vi "goToVf.vi"(9 "RobotModelAllInformation in":T1, 10 "firstCall?":bool, 11 "Robot in":refnum<class "Robot.lvclass">) -> (2 "RobotModelAllInformation out":T1, 3 "Robot out":refnum<class "Robot.lvclass">)   [LabVIEW 2020, in "Game.lvclass"]
uses:
  Game.lvclass
  Controls/RobotModel.ctl
  Controls/RobotModelAllInformation.ctl
  Controls/RobotModelTestCrashCase.ctl
  Robot_class/Robot.lvclass
  C:/RoboIME/SSL_AI/Object_class/Object.lvclass
  Robot_class/Robot.lvclass/Robot.ctl
  Object_class/Object.lvclass/Object.ctl
  <vilib>/Analysis/_algsub.llb/Real Vector Norm.vi
  Object_class/Read x.vi
  Object_class/Read y.vi
  Robot_class/Read est_v_tang.vi
  Robot_class/Write v_tang.vi
  Robot_class/Write v_norm.vi
  Robot_class/Write v_ang.vi
  <vilib>/Analysis/NI_AALPro.lvlib
panel:
  in  "RobotModel":T2
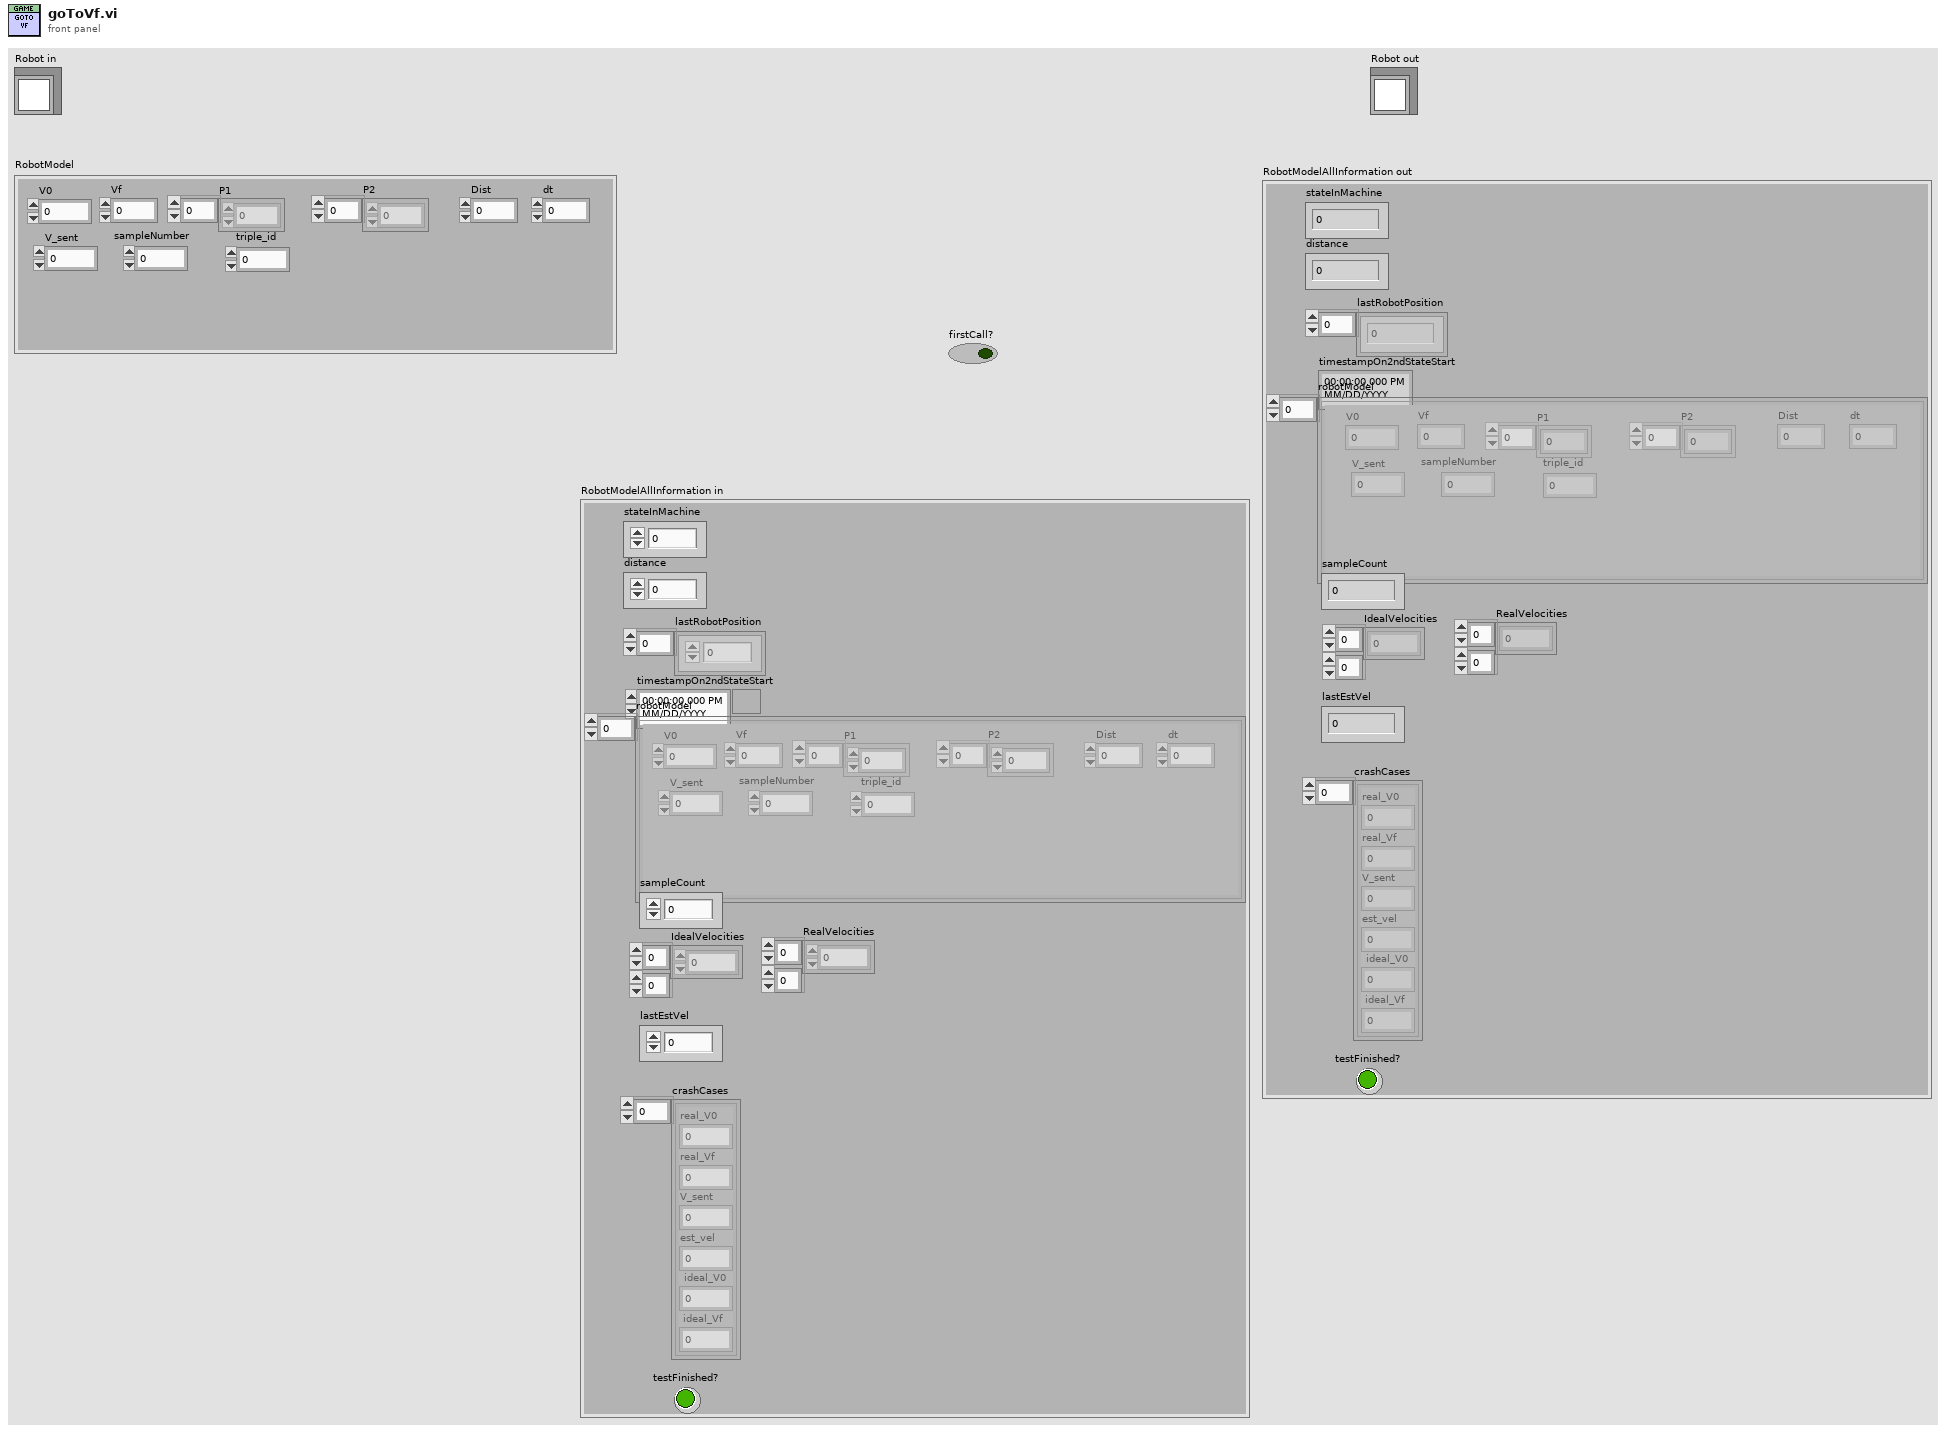
[diagram p1: front panel]
types:
  T1 = typedef "RobotModelAllInformation.ctl" = cluster{"distance":dbl, "lastRobotPosition":dbl[], "timestampOn2ndStateStart":timestamp, "robotModel":T2[], "sampleCount":i32, "stateInMachine":i32, "crashCases":T3[], "lastEstVel":dbl, "IdealVelocities":dbl[][], "RealVelocities":dbl[][], "testFinished?":bool}
  T2 = typedef "RobotModel.ctl" = cluster{"V0":dbl, "Vf":dbl, "Dist":dbl, "dt":dbl, "P1":dbl[], "P2":dbl[], "V_sent":dbl, "sampleNumber":i32, "triple_id":i32}
  T3 = typedef "RobotModelTestCrashCase.ctl" = cluster{"real_V0":dbl, "real_Vf":dbl, "V_sent":dbl, "est_vel":dbl, "ideal_V0":dbl, "ideal_Vf":dbl}
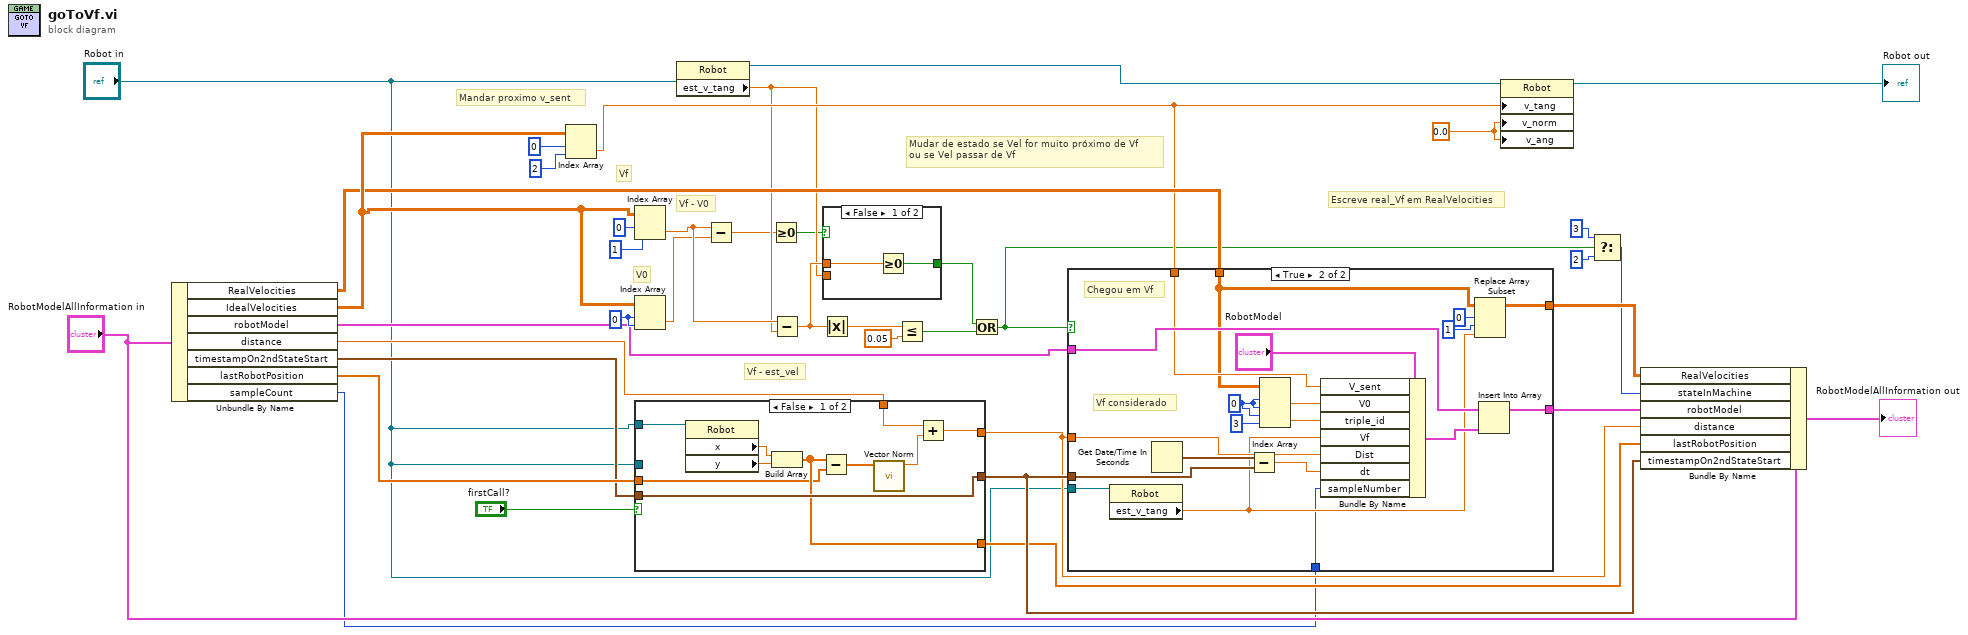
[diagram p0: block diagram]
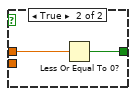
[diagram p2: hidden frame]
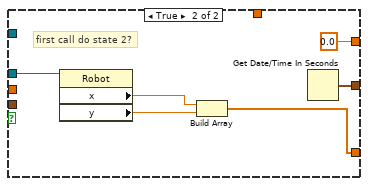
[diagram p4: hidden frame]
diagram:
  w38 = 0 ("index (row)")
  w3 = 0.0 ("v_norm")
  # "Escreve real_Vf em RealVelocities"
  # "Vf - est_vel"
  # "V0"
  # "Vf"
  # "Vf - V0"
  # "Mandar proximo v_sent"
  # "Mudar de estado se Vel for muito próximo de Vf\nou se Vel passar de Vf"
  n1 = Unbundle By Name("RobotModelAllInformation in") -> ("RealVelocities"=w29:dbl[][], "IdealVelocities"=w37:dbl[][], "robotModel"=w21:T2[], "distance"=w32:dbl, "timestampOn2ndStateStart"=w24:timestamp, "lastRobotPosition"=w30:dbl[], "sampleCount"=w1:i32)
  n2 = Index Array(array=w37, index (row)=0, index (col)=2 ("disabled index (col)")) -> (element=w28:dbl)
  n3 = Index Array(array=w37, index (row)=0, index (col)=1 ("disabled index (col)")) -> (element=w36:dbl)
  n4 = Index Array(array=w37, index (row)=w38, index (col)=w38) -> (element=w10:dbl)
  n5 = case shown="False" "firstCall?" {
    tunnel: [w49 w55] -> w33
    tunnel: w24 -> [w49 _]
    tunnel: "Robot in" -> [_ w54]
    tunnel: "Robot in" -> [w46 _]
    tunnel: [w40 0.0] -> w31
    tunnel: [w45 w51] -> w23
    tunnel: w30 -> [w43 _]
    tunnel: w32 -> [w42 _]
    frame False {
      n6 = property class="Robot"(reference=w46) -> ("x"=w47:dbl, "y"=w48:dbl)  [unwired: 1 in, 2 out]
      n7 = Build Array(w47, w48) -> (w45:dbl[])
      n8 = Subtract(x=w45, y=w43) -> (x-y=w44:dbl[])
      n9 = call-poly <vilib>:"Vector Norm.vi"("Input Vector"=w44) -> ("norm"=w41:dbl)  [unwired: 9 in, 1 out]
      n10 = Add(x=w42, y=w41) -> (x+y=w40:dbl)
    }
    frame True {
      # "first call do state 2?"
      n11 = property class="Robot"(reference=w54) -> ("x"=w53:dbl, "y"=w52:dbl)  [unwired: 1 in, 2 out]
      n12 = Build Array(w53, w52) -> (w51:dbl[])
      n13 = Get Date/Time In Seconds() -> (seconds since 1Jan1904=w55:timestamp)
    }
  }
  n14 = property class="Robot"(reference="Robot in") -> (reference out=w4:refnum<class "Robot.lvclass">, "est_v_tang"=w12:dbl)  [unwired: 1 in, 1 out]
  n15 = Subtract(x=w36, y=w10) -> (x-y=w7:dbl)
  n16 = Greater Or Equal To 0?(x=w7) -> (x >= 0?=w9:bool)
  n17 = Subtract(x=w36, y=w12) -> (x-y=w13:dbl)
  n18 = Absolute Value(x=w13) -> (abs(x)=w14:dbl)
  n19 = case shown="False" w9 {
    tunnel: [w57 w59] -> w16
    tunnel: w12 -> [_ _]
    tunnel: w13 -> [w56 w58]
    frame False {
      n20 = Greater Or Equal To 0?(x=w56) -> (x >= 0?=w57:bool)
    }
    frame True {
      n21 = Less Or Equal To 0?(x=w58) -> (x <= 0?=w59:bool)
    }
  }
  n22 = Less Or Equal?(x=w14, y=0.05) -> (x <= y?=w15:bool)
  n23 = Or(x=w16, y=w15) -> (x .or. y?=w17:bool)
  n24 = case shown="True" w17 {
    tunnel: "Robot in" -> [_ w80]
    tunnel: w21 -> [w61 w76]
    tunnel: [w61 w74] -> w22
    tunnel: w33 -> [_ w78]
    tunnel: w31 -> [_ w72]
    tunnel: w28 -> [_ w71]
    tunnel: w29 -> [w60 w70]
    tunnel: [w60 w67] -> w39
    tunnel: w1 -> [_ w65]
    frame False {
    }
    frame True {
      w64 = 0 ("index (row)")
      # "Vf considerado"
      # "Chegou em Vf"
      n25 = property class="Robot"(reference=w80) -> ("est_v_tang"=w66:dbl)  [unwired: 1 in, 2 out]
      n26 = Get Date/Time In Seconds() -> (seconds since 1Jan1904=w79:timestamp)
      n27 = Subtract(x=w79, y=w78) -> (x-y=w77:dbl)
      n28 = Index Array(array=w70, index (row) #1=w64, index (col) #1=w64, index (row) #2=w64, index (col) #2=3 ("disabled index (col)")) -> (element #1=w81:dbl, element #2=w62:dbl)
      n29 = Bundle By Name(cluster="RobotModel", "V_sent"=w71, "V0"=w81, "triple_id"=w62, "Vf"=w66, "Dist"=w72, "dt"=w77, "sampleNumber"=w65) -> (w75:T2)
      n30 = Replace Array Subset(array=w70, new element=w66, index (row)=0, index (col)=1 ("disabled index (col)")) -> (w67:dbl[][])
      n31 = Insert Into Array(array=w76, new element=w75) -> (w74:T2[])  [unwired: 1 in]
    }
  }
  n32 = property class="Robot"(reference=w4, "v_tang"=w28, "v_norm"=w3, "v_ang"=w3) -> (reference out=→"Robot out":refnum<class "Robot.lvclass">)  [unwired: 1 in, 1 out]
  n33 = Select(t=3, s=w17, f=2) -> (s? t:f=w19:i32)
  n34 = Bundle By Name(cluster="RobotModelAllInformation in", "RealVelocities"=w39, "stateInMachine"=w19, "robotModel"=w22, "distance"=w31, "lastRobotPosition"=w23, "timestampOn2ndStateStart"=w33) -> (→"RobotModelAllInformation out":T1)
